vi "5pt Mov Avg.vi"(10 "Value in":dbl) -> (2 "Value out":dbl)   [LabVIEW 2014]
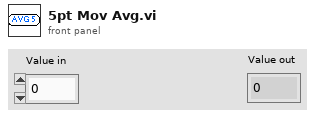
[diagram p1: front panel]
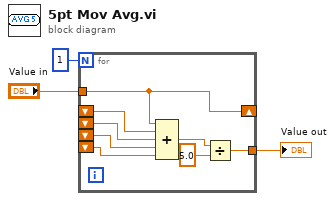
[diagram p0: block diagram]
diagram:
  n1 = for {
    N: 1 -> [_]
    tunnel: "Value in" -> [w11]
    shift-right: [w11] -> _
    shift-left: _ -> [w10]
    shift-left: _ -> [w9]
    tunnel: [w6] -> w1
    shift-left: _ -> [w5]
    shift-left: _ -> [w4]
    n2 = Compound Arithmetic op=ADD(w11, w10, w9, w5, w4) -> (w8:dbl)
    n3 = Divide(x=w8, y=5.0) -> (x/y=w6:dbl)
  }
  "Value out" <- w1
